vi "Write Return Devices to Load IDs Msg.vi"(10 "Return Devices to Load IDs Msg":refnum<class "Return Devices to Load IDs Msg.lvclass">, 11 "Devices to Load in":refnum<class "Devices to Load.lvclass">) -> (3 "Devices to Load out":refnum<class "Devices to Load.lvclass">)   [LabVIEW 2018, in "Devices to Load Config Actor.lvlib" / "Devices to Load.lvclass"]
uses:
  Devices to Load.lvclass
  Devices to Load Messages/Return Devices to Load IDs Msg/Return Devices to Load IDs Msg.lvclass
  Devices to Load.lvclass/Devices to Load.ctl
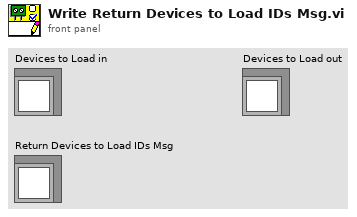
[diagram p1: front panel]
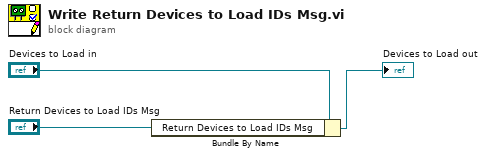
[diagram p0: block diagram]
diagram:
  n1 = Bundle By Name(cluster="Devices to Load in", "Return Devices to Load IDs Msg"="Return Devices to Load IDs Msg") -> (→"Devices to Load out":refnum<class "Devices to Load.lvclass">)
